vi "Stop Core.vi"(10 "final error code":i32, 11 "BNT_DAQmx-MCSV-DOPWM in":refnum<class "BNT_DAQmx-MCSV-DOPWM.lvclass">) -> (3 "BNT_DAQmx-MCSV-DOPWM out":refnum<class "BNT_DAQmx-MCSV-DOPWM.lvclass">)   [LabVIEW 2017, in "BNT_DAQmx.lvlib" / "BNT_DAQmx-MCSV-DOPWM.lvclass"]
doc: "(<B>Filename</B>: Actor Framework.lvlib:Actor.lvclass:Stop Core.vi)\n\nDefines what the actor does before it stops. Use the <B>final error code</B> input to determine whether the actor shut down in response to an error.\n\nBy default, this method does nothing. A descendant class may override it to define behavior, such as shutting down any processes the actor initiated in its override of the Actor Core method."
uses:
  BNT_DAQmx-MCSV-DOPWM.lvclass
  BNT_DAQmx-MCSV-DOPWM.lvclass/BNT_DAQmx-MCSV-DOPWM.ctl
  BNT_DAQmx-MCSV/BNT_DAQmx-MCSV.lvclass
  CSPP_Core/Classes/CSPP_ProcessVariables/PVConnection/PVConnection.lvclass
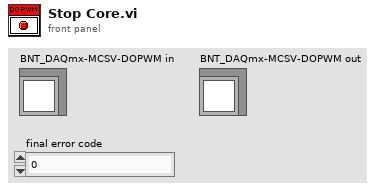
[diagram p1: front panel]
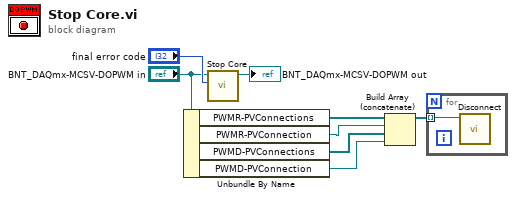
[diagram p0: block diagram]
diagram:
  n1 = Unbundle By Name("BNT_DAQmx-MCSV-DOPWM in") -> ("PWMR-PVConnections"=w5:refnum<class "PVConnection.lvclass">[], "PWMR-PVConnection"=w3:refnum<class "PVConnection.lvclass">, "PWMD-PVConnections"=w2:refnum<class "PVConnection.lvclass">[], "PWMD-PVConnection"=w1:refnum<class "PVConnection.lvclass">)
  n2 = call-parent "Stop Core.vi"("final error code"="final error code", "BNT_DAQmx-MCSV in"="BNT_DAQmx-MCSV-DOPWM in") -> ("BNT_DAQmx-MCSV out"=→"BNT_DAQmx-MCSV-DOPWM out":refnum<class "BNT_DAQmx-MCSV-DOPWM.lvclass">)  [unwired: 9 in]
  n3 = Build Array (concatenate)(w5, w3, w2, w1) -> (w4:refnum<class "PVConnection.lvclass">[])
  n4 = for {
    tunnel: w4 -> [w9] mode=indexing
    n5 = call "Disconnect.vi"("PVConnection in"=w9) -> ()  [unwired: 9 in, 2 out]
  }
